vi "Run_Pre Core.vi"(0 "While Loop in":refnum<class "Structure Loop.lvclass">, 11 "error in (no error)":errorcluster) -> (4 "While Loop out":refnum<class "Structure Loop.lvclass">, 6 "Execute Run Core?":bool, 15 "error out":errorcluster)   [LabVIEW 2016, in "Structure Loop.lvclass"]
uses:
  Structure Loop.lvclass
  Structure Loop.lvclass/Structure Loop.ctl
  functionsbase/functionbase.lvclass
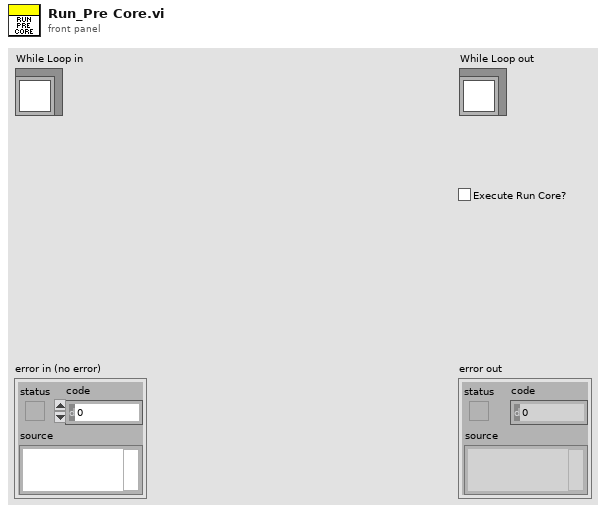
[diagram p1: front panel]
types:
  T1 = typedef "Structure Loop.lvclass/Function List.ctl" = enum16{"For Loop", "While Loop"}
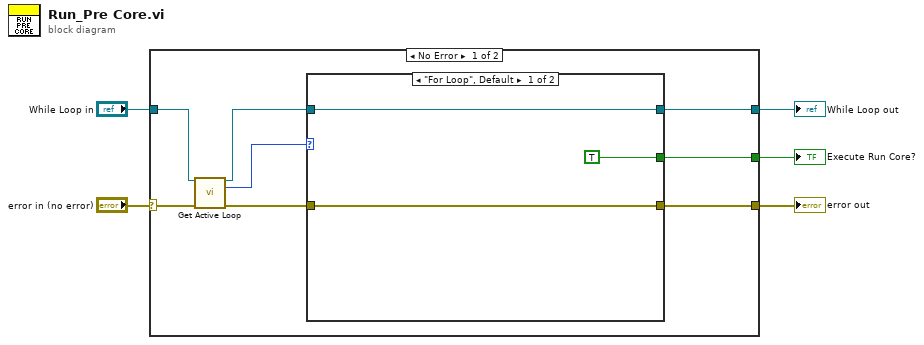
[diagram p0: block diagram]
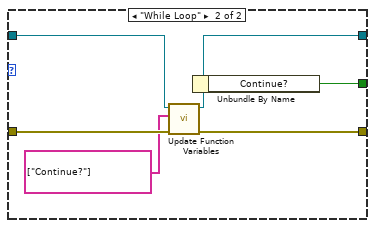
[diagram p2: hidden frame]
diagram:
  n1 = case shown="No Error" "error in (no error)" {
    selector: "error in (no error)" -> [w10 w24]
    tunnel: "While Loop in" -> [w8 w23]
    tunnel: [w13 _] -> w4
    tunnel: [w11 w23] -> w3
    tunnel: [w12 w24] -> w1
    frame No Error {
      n2 = call "Get Active Loop.vi"("Structure Loop in"=w8, "error in (no error)"=w10) -> ("Structure Loop out"=w7:refnum<class "Structure Loop.lvclass">, "Function List"=w6:T1, "error out"=w9:errorcluster)  [unwired: 11 in]
      n3 = case shown="\"For Loop\", Default" w6 {
        tunnel: [TRUE ("Continue?") w22] -> w13
        tunnel: [w14 w21] -> w12
        tunnel: [w16 w20] -> w11
        tunnel: w9 -> [w14 w19]
        tunnel: w7 -> [w16 w18]
        frame "For Loop", Default {
        }
        frame "While Loop" {
          n4 = call "Update Function Variables.vi"("error in (no error)"=w19, "Variable Names"=string[] ["Continue?"], "Structure Loop in"=w18) -> ("error out"=w21:errorcluster, "Structure Loop out"=w20:refnum<class "Structure Loop.lvclass">)  [unwired: 7 in]
          n5 = Unbundle By Name(w20) -> ("Continue?"=w22:bool)
        }
      }
    }
    frame Error {
    }
  }
  "error out" <- w1
  "While Loop out" <- w3
  "Execute Run Core?" <- w4
